vi "Inficon Hot Water Calculation.vi"(7 "RTD Out (°F)":dbl, 8 "Error In":errorcluster, 11 "Emerson Flow Meter Data Output":T1) -> (0 "Error Out":errorcluster, 3 "Emerson Flow Meter Data Output 2":T1)   [LabVIEW 2019]
uses:
  Type Definitions/Inficon Data.ctl
panel:
  # "Natural Gas"
  # "Propane"
  # "Natural Gas"
  # "Propane"
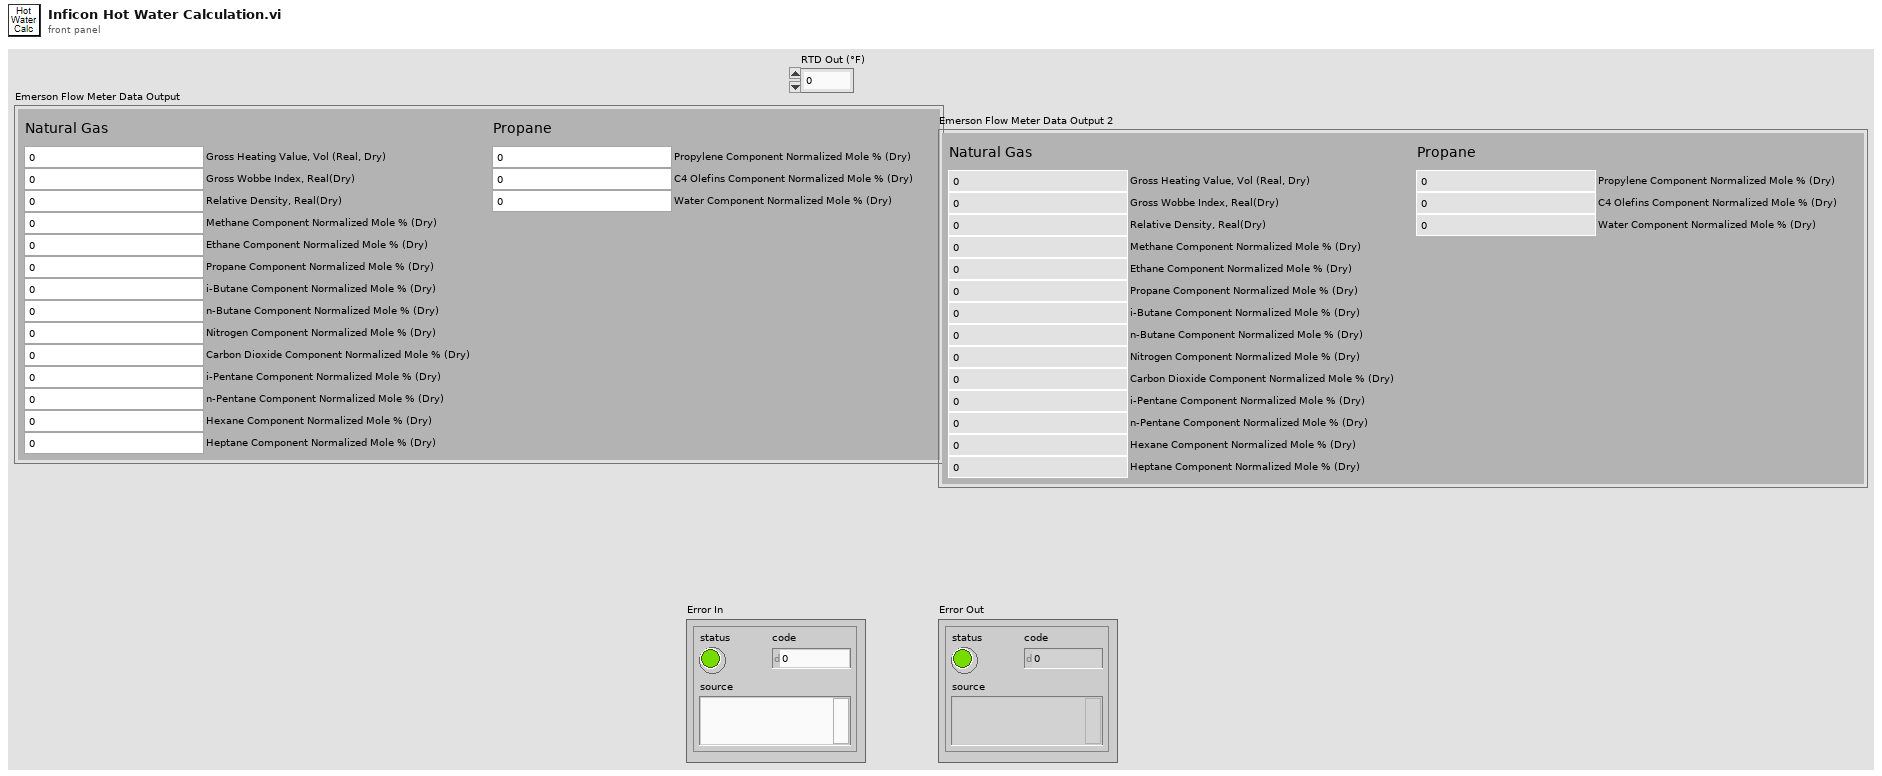
[diagram p1: front panel]
types:
  T1 = typedef "Inficon Data.ctl" = cluster{"Gross Heating Value, Vol (Real, Dry)":dbl, "Nitrogen Component Normalized Mole % (Dry)":dbl, "Methane Component Normalized Mole % (Dry)":dbl, "Carbon Dioxide Component Normalized Mole % (Dry)":dbl, "Ethane Component Normalized Mole % (Dry)":dbl, "Propane Component Normalized Mole % (Dry)":dbl, "i-Pentane Component Normalized Mole % (Dry)":dbl, "i-Butane Component Normalized Mole % (Dry)":dbl, "n-Butane Component Normalized Mole % (Dry)":dbl, "n-Pentane Component Normalized Mole % (Dry)":dbl, "Hexane Component Normalized Mole % (Dry)":dbl, "Heptane Component Normalized Mole % (Dry)":dbl, "Gross Wobbe Index, Real(Dry)":dbl, "Relative Density, Real(Dry)":dbl, "Propylene Component Normalized Mole % (Dry)":dbl, "C4 Olefins Component Normalized Mole % (Dry)":dbl, "Water Component Normalized Mole % (Dry)":dbl}
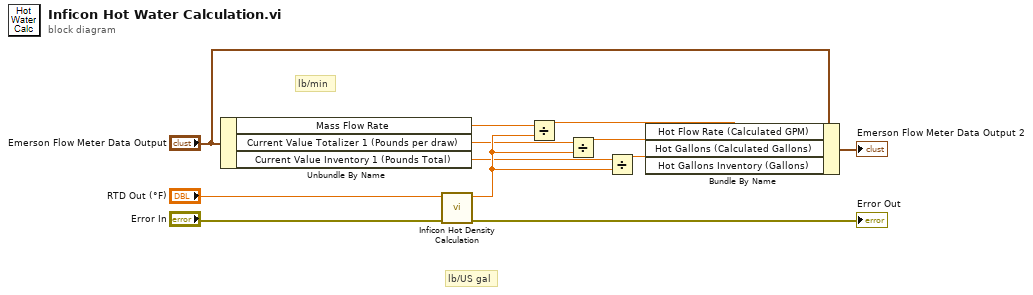
[diagram p0: block diagram]
diagram:
  # "lb/min"
  # "lb/US gal"
  n1 = Unbundle By Name("Emerson Flow Meter Data Output") -> ("Mass Flow Rate"=w10:dbl, "Current Value Totalizer 1 (Pounds per draw)"=w4:dbl, "Current Value Inventory 1 (Pounds Total)"=w3:dbl)
  n2 = call "Inficon Hot Density Calculation.vi"("Error In"="Error In", "RTD Out (°F)"="RTD Out (°F)") -> ("Error Out"=→"Error Out":errorcluster, "Density (lb/gal)"=w5:dbl)  [unwired: 8 in]
  n3 = Divide(x=w10, y=w5) -> (x/y=w8:dbl)
  n4 = Divide(x=w4, y=w5) -> (x/y=w2:dbl)
  n5 = Divide(x=w3, y=w5) -> (x/y=w1:dbl)
  n6 = Bundle By Name(cluster="Emerson Flow Meter Data Output", "Hot Flow Rate (Calculated GPM)"=w8, "Hot Gallons (Calculated Gallons)"=w2, "Hot Gallons Inventory (Gallons)"=w1) -> (→"Emerson Flow Meter Data Output 2":T1)
